vi "log analysis_gps.vi"() -> ()   [LabVIEW 2018] (continued)
0.0,0.000000000,0.000000000,\"631T\",11,3,3,3,04,00,20,00*7e5de74c\n\tsystem status\tnormal 2 27.700000 0 0\trobot status\t45.202909\t59.882712\t8.918700\t-0.461335\t0.674834\t-123.113809\t0.488000\t0.005000\n\t\n15:51:02.4\tlog_raw\tgps_raw\t#INSPVAXA,USB3,0,53.0,FINESTEERING,2107,283880.400,02000000,471d,15824;INS_ALIGNMENT_COMPLETE,INS_RTKFIXED,37.37066797060,126.72134375029,8.9215,22.3000,-0.3538,-0.2783,0.0388,-0.597615608,0.513014169,213.355161065,0.4357,0.3062,0.6023,0.1133,0.0940,0.0839,0.0973,0.1012,5.1494,0f000001,0*cddeff4e\n\tsystem status\tnormal 2 27.800000 0 0\trobot status\t45.054959\t59.684519\t8.921500\t-0.597616\t0.513014\t-123.355161\t0.488000\t-0.003000\n\t\n15:51:02.9\tlog_raw\tgps_raw\t#INSPVAXA,USB3,0,53.0,FINESTEERING,2107,283880.900,02000000,471d,15824;INS_ALIGNMENT_COMPLETE,INS_RTKFIXED,37.37066635165,126.72134221442,8.9278,22.3000,-0.3658,-0.2852,0.0396,-0.626245150,0.597396810,213.371902809,0.4357,0.3062,0.6023,0.1133,0.0940,0.0839,0.0973,0.1012,5.1494,0f000001,0*bdd5d949\n\tsystem status\tnormal 2 27.700000 0 0\trobot status\t44.918914\t59.504842\t8.927800\t-0.626245\t0.597397\t-123.371903\t0.492000\t0.000000\n\t\n15:51:03.4\tlog_raw\tgps_raw\t#DUALANTENNAHEADINGA,USB3,0,50.5,FINESTEERING,2107,283881.400,02000000,d426,15824;INSUFFICIENT_OBS,NONE,-1.000000000,0.000000000,0.000000000,0.0,0.000000000,0.000000000,\"631T\",11,3,3,3,04,00,20,00*4d958a84\n\tsystem status\tnormal 2 27.800000 0 0\trobot status\t44.773617\t59.313122\t8.931900\t-0.646552\t0.444640\t-123.445577\t0.501000\t0.006000\n\t\n15:51:03.9\tlog_raw\tgps_raw\t#INSPVAXA,USB3,0,50.5,FINESTEERING,2107,283881.900,02000000,471d,15824;INS_ALIGNMENT_COMPLETE,INS_RTKFIXED,37.37066299197,126.72133897955,8.9361,22.3000,-0.3474,-0.2868,0.0393,-0.593672744,0.610910921,213.511371032,0.4358,0.3048,0.6020,0.1139,0.0948,0.0841,0.0973,0.1012,5.1504,0f000001,0*060d8030\n\tsystem status\tnormal 2 27.700000 0 0\trobot status\t44.632374\t59.131970\t8.936100\t-0.593673\t0.610911\t-123.511371\t0.482000\t-0.001000\n\t\n15:51:04.4\tlog_raw\tgps_raw\t#DUALANTENNAHEADINGA,USB3,0,51.5,FINESTEERING,2107,283882.400,02000000,d426,15824;INSUFFICIENT_OBS,NONE,-1.000000000,0.000000000,0.000000000,0.0,0.000000000,0.000000000,\"631T\",12,3,3,3,04,00,20,00*3cefd7e2\n\tsystem status\tnormal 2 27.800000 0 0\trobot status\t44.487766\t58.944941\t8.939800\t-0.440117\t0.780812\t-123.484878\t0.511000\t0.000000\n\t\n15:51:04.9\tlog_raw\tgps_raw\t#INSPVAXA,USB3,0,51.5,FINESTEERING,2107,283882.900,02000000,471d,15824;INS_ALIGNMENT_COMPLETE,INS_RTKFIXED,37.37065963052,126.72133572900,8.9416,22.3000,-0.3499,-0.2875,0.0236,-0.546470396,0.861326947,213.517075808,0.4357,0.3040,0.6014,0.1142,0.0952,0.0840,0.0973,0.1012,5.1519,0f000001,0*24ce4552\n\tsystem status\tnormal 2 27.800000 0 0\trobot status\t44.344446\t58.758903\t8.941600\t-0.546470\t0.861327\t-123.517076\t0.491000\t-0.002000\n\t\n15:51:05.4\tlog_raw\tgps_raw\t#INSPVAXA,USB3,0,52.0,FINESTEERING,2107,283883.400,02000000,471d,15824;INS_ALIGNMENT_COMPLETE,INS_RTKFIXED,37.37065796164,126.72133411405,8.9451,22.3000,-0.3685,-0.2983,0.0398,-0.521036438,0.724479041,213.604247881,0.4353,0.3043,0.6007,0.1142,0.0953,0.0836,0.0972,0.1012,5.1533,0f000001,0*63d3ff51\n\tsystem status\tnormal 2 27.800000 0 0\trobot status\t44.201396\t58.573683\t8.945100\t-0.521036\t0.724479\t-123.604248\t0.493000\t-0.004000\n\t\n15:51:05.9\tlog_raw\tgps_raw\t#DUALANTENNAHEADINGA,USB3,0,52.0,FINESTEERING,2107,283883.900,02000000,d426,15824;INSUFFICIENT_OBS,NONE,-1.000000000,0.000000000,0.000000000,0.0,0.000000000,0.000000000,\"631T\",10,3,3,3,04,00,20,00*65cb768f\n\tsystem status\tnormal 2 27.800000 0 0\trobot status\t44.054708\t58.385576\t8.946000\t-0.360090\t0.706848\t-123.677696\t0.503000\t-0.011000\n\t\n15:51:06.4\tlog_raw\tgps_raw\t#DUALANTENNAHEADINGA,USB3,0,49.5,FINESTEERING,2107,283884.400,02000000,d426,15824;INSUFFICIENT_OBS,NONE,-1.000000000,0.000000000,0.000000000,0.0,0.000000000,0.000000000,\"631T\",9,3,3,3,04,00,20,00*1d3e0ccf\n\tsystem status\tnormal 2 27.800000 0 0\trobot status\t43.913169\t58.198898\t8.948900\t-0.506488\t0.685418\t-123.687701\t0.497000\t0.009000\n\t\n15:51:06.9\tlog_raw\tgps_raw\t#DUALANTENNAHEADINGA,USB3,0,49.5,FINESTEERING,2107,283884.900,02000000,d426,15824;INSUFFICIENT_OBS,NONE,-1.000000000,0.000000000,0.000000000,0.0,0.000000000,0.000000000,\"631T\",10,3,3,3,04,00,20,00*031e6964\n\tsystem status\tnormal 2 27.700000 0 0\trobot status\t43.771695\t58.014475\t8.953600\t-0.483140\t0.799105\t-123.568013\t0.566000\t-0.106000\n\t\n15:51:07.4\tlog_raw\tgps_raw\t#INSPVAXA,USB3,0,51.5,FINESTEERING,2107,283885.400,02000000,471d,15824;INS_ALIGNMENT_COMPLETE,INS_RTKFIXED,37.37065120654,126.72132762399,8.9567,22.3000,-0.3599,-0.3036,0.0416,-0.421250384,0.704031349,213.500996788,0.4347,0.3046,0.5988,0.1136,0.0944,0.0821,0.0969,0.1010,5.1559,0f000001,0*f6e8d8e3\n\tsystem status\tnormal 2 27.800000 0 0\trobot status\t43.626517\t57.823974\t8.956700\t-0.421250\t0.704031\t-123.500997\t0.476000\t0.038000\n\t\n15:51:07.9\tlog_raw\tgps_raw\t#DUALANTENNAHEADINGA,USB3,0,51.5,FINESTEERING,2107,283885.900,02000000,d426,15824;INSUFFICIENT_OBS,NONE,-1.000000000,0.000000000,0.000000000,0.0,0.000000000,0.000000000,\"631T\",9,3,3,3,04,00,20,00*45f2a281\n\tsystem status\tnormal 2 27.700000 0 0\trobot status\t43.483999\t57.637312\t8.961400\t-0.525632\t0.753190\t-123.406586\t0.428000\t0.092000\n\t\n15:51:08.4\tlog_raw\tgps_raw\t#DUALANTENNAHEADINGA,USB3,0,53.0,FINESTEERING,2107,283886.400,02000000,d426,15824;INSUFFICIENT_OBS,NONE,-1.000000000,0.000000000,0.000000000,0.0,0.000000000,0.000000000,\"631T\",9,3,3,3,04,00,20,00*f304b34d\n\tsystem status\tnormal 2 27.700000 0 0\trobot status\t43.341734\t57.449911\t8.964400\t-0.655210\t0.560645\t-123.324017\t0.473000\t0.021000\n\t\n15:51:08.9\tlog_raw\tgps_raw\t#DUALANTENNAHEADINGA,USB3,0,53.0,FINESTEERING,2107,283886.900,02000000,d426,15824;INSUFFICIENT_OBS,NONE,-1.000000000,0.000000000,0.000000000,0.0,0.000000000,0.000000000,\"631T\",9,3,3,3,04,00,20,00*6aeedf3b\n\tsystem status\tnormal 2 27.800000 0 0\trobot status\t43.199784\t57.262939\t8.968200\t-0.680653\t0.754053\t-123.210428\t0.466000\t0.053000\n\t\n15:51:09.4\tlog_raw\tgps_raw\t#DUALANTENNAHEADINGA,USB3,0,53.0,FINESTEERING,2107,283887.400,02000000,d426,15824;INSUFFICIENT_OBS,NONE,-1.000000000,0.000000000,0.000000000,0.0,0.000000000,0.000000000,\"631T\",9,3,3,3,04,00,20,00*f6e48158\n\tsystem status\tnormal 2 27.700000 0 0\trobot status\t43.057634\t57.072018\t8.971600\t-0.763083\t0.466087\t-123.102293\t0.415000\t0.111000\n\t\n15:51:09.9\tlog_raw\tgps_raw\t#DUALANTENNAHEADINGA,USB3,0,53.0,FINESTEERING,2107,283887.900,02000000,d426,15824;INSUFFICIENT_OBS,NONE,-1.000000000,0.000000000,0.000000000,0.0,0.000000000,0.000000000,\"631T\",9,3,3,3,04,00,20,00*6f0eed2e\n\tsystem status\tnormal 2 27.800000 0 0\trobot status\t42.915933\t56.883397\t8.974500\t-0.641098\t0.390257\t-123.007682\t0.428000\t0.084000\n\t\n15:51:10.4\tlog_raw\tgps_raw\t#DUALANTENNAHEADINGA,USB3,0,52.5,FINESTEERING,2107,283888.400,02000000,d426,15824;INSUFFICIENT_OBS,NONE,-1.000000000,0.000000000,0.000000000,0.0,0.000000000,0.000000000,\"631T\",10,3,3,3,04,00,20,00*e7048907\n\tsystem status\tnormal 2 27.700000 0 0\trobot status\t42.775640\t56.696889\t8.979100\t-0.681003\t0.747105\t-122.877604\t0.588000\t-0.127000\n\t\n15:51:10.9\tlog_raw\tgps_raw\t#DUALANTENNAHEADINGA,USB3,0,52.5,FINESTEERING,2107,283888.900,02000000,d426,15824;INSUFFICIENT_OBS,NONE,-1.000000000,0.000000000,0.000000000,0.0,0.000000000,0.000000000,\"631T\",10,3,3,3,04,00,20,00*5efbb762\n\tsystem status\tnormal 2 27.700000 0 0\trobot status\t42.634078\t56.507649\t8.981700\t-0.814755\t0.597074\t-122.710020\t0.592000\t-0.135000\n\t\n15:51:11.4\tlog_raw\tgps_raw\t#DUALANTENNAHEADINGA,USB3,0,46.0,FINESTEERING,2107,283889.400,02000000,d426,15824;INSUFFICIENT_OBS,NONE,-1.000000000,0.000000000,0.000000000,0.0,0.000000000,0.000000000,\"631T\",11,3,3,3,04,00,20,00*93f994bc\n\tsystem status\tnormal 2 27.700000 0 0\trobot status\t42.495049\t56.319089\t8.986300\t-0.601073\t0.725458\t-122.679569\t0.468000\t0.025000\n\t\n15:51:11.9\tlog_raw\tgps_raw\t#DUALANTENNAHEADINGA,USB3,0,46.0,FINESTEERING,2107,283889.900,02000000,d426,15824;INSUFFICIENT_OBS,NONE,-1.000000000,0.000000000,0.000000000,0.0,0.000000000,0.000000000,\"631T\",11,3,3,3,04,00,20,00*2a06aad9\n\tsystem status\tnormal 2 27.800000 0 0\trobot status\t42.353484\t56.121425\t8.991300\t-0.835162\t0.704682\t-122.703827\t0.503000\t-0.001000\n\t\n15:51:12.4\tlog_raw\tgps_raw\t#DUALANTENNAHEADINGA,USB3,0,49.5,FINESTEERING,2107,283890.400,02000000,d426,15824;INSUFFICIENT_OBS,NONE,-1.000000000,0.000000000,0.000000000,0.0,0.000000000,0.000000000,\"631T\",11,3,3,3,04,00,20,00*fe707008\n\tsystem status\tnormal 2 27.800000 0 0\trobot status\t42.214536\t55.932405\t8.994000\t-0.832597\t0.803383\t-122.691479\t0.495000\t-0.002000\n\t\n15:51:12.9\tlog_raw\tgps_raw\t#DUALANTENNAHEADINGA,USB3,0,49.5,FINESTEERING,2107,283890.900,02000000,d426,15824;INSUFFICIENT_OBS,NONE,-1.000000000,0.000000000,0.000000000,0.0,0.000000000,0.000000000,\"631T\",11,3,3,3,04,00,20,00*478f4e6d\n\tsystem status\tnormal 2 27.800000 0 0\trobot status\t42.072498\t55.741837\t8.997200\t-0.759363\t0.656487\t-122.762965\t0.579000\t-0.139000\n\t\n15:51:13.4\tlog_raw\tgps_raw\t#DUALANTENNAHEADINGA,USB3,0,50.5,FINESTEERING,2107,283891.400,02000000,d426,15824;INSUFFICIENT_OBS,NONE,-1.000000000,0.000000000,0.000000000,0.0,0.000000000,0.000000000,\"631T\",12,3,3,3,04,00,20,00*11a1be59\n\tsystem status\tnormal 2 27.700000 0 0\trobot status\t41.933995\t55.549806\t9.002300\t-0.915873\t0.288769\t-122.684066\t0.471000\t0.023000\n\t\n15:51:13.9\tlog_raw\tgps_raw\t#DUALANTENNAHEADINGA,USB3,0,50.5,FINESTEERING,2107,283891.900,02000000,d426,15824;INSUFFICIENT_OBS,NONE,-1.000000000,0.000000000,0.000000000,0.0,0.000000000,0.000000000,\"631T\",11,3,3,3,04,00,20,00*0b080695\n\tsystem status\tnormal 2 27.800000 0 0\trobot status\t41.790012\t55.354180\t9.005600\t-0.810761\t0.437065\t-122.626399\t0.585000\t-0.144000\n\t\n15:51:14.4\tlog_raw\tgps_raw\t#DUALANTENNAHEADINGA,USB3,0,51.0,FINESTEERING,2107,283892.400,02000000,d426,15824;INSUFFICIENT_OBS,NONE,-1.000000000,0.000000000,0.000000000,0.0,0.000000000,0.000000000,\"631T\",12,3,3,3,04,00,20,00*96f7835a\n\tsystem status\tnormal 2 27.800000 0 0\trobot status\t41.651158\t55.165638\t9.008000\t-0.628580\t0.466952\t-122.705405\t0.519000\t-0.026000\n\t\n15:51:14.9\tlog_raw\tgps_raw\t#DUALANTENNAHEADINGA,USB3,0,51.0,FINESTEERING,2107,283892.900,02000000,d426,15824;INSUFFICIENT_OBS,NONE,-1.000000000,0.000000000,0.000000000,0.0,0.000000000,0.000000000,\"631T\",11,3,3,3,04,00,20,00*8c5e3b96\n\tsystem status\tnormal 2 27.800000 0 0\trobot status\t41.510596\t54.974116\t9.012100\t-0.618825\t0.500579\t-122.716893\t0.486000\t0.000000\n\t\n15:51:15.4\tlog_raw\tgps_raw\t#DUALANTENNAHEADINGA,USB3,0,50.5,FINESTEERING,2107,283893.400,02000000,d426,15824;INSUFFICIENT_OBS,NONE,-1.000000000,0.000000000,0.000000000,0.0,0.000000000,0.000000000,\"631T\",12,3,3,3,04,00,20,00*ca11b7eb\n\tsystem status\tnormal 2 27.800000 0 0\trobot status\t41.369608\t54.781650\t9.014800\t-0.929782\t0.617797\t-122.679558\t0.590000\t-0.141000\n\t\n15:51:15.9\tlog_raw\tgps_raw\t#INSPVAXA,USB3,0,50.5,FINESTEERING,2107,283893.900,02000000,471d,15824;INS_ALIGNMENT_COMPLETE,INS_RTKFIXED,37.37062209490,126.72130052647,9.0192,22.3000,-0.3742,-0.3207,0.0346,-0.662095727,0.862366850,212.722532448,0.4356,0.3043,0.5955,0.1140,0.0944,0.0837,0.0963,0.1003,5.1649,0f000001,0*3a5d3b07\n\tsystem status\tnormal 2 27.800000 0 0\trobot status\t41.226263\t54.593043\t9.019200\t-0.662096\t0.862367\t-122.722532\t0.512000\t-0.016000\n\t\n15:51:16.4\tlog_raw\tgps_raw\t#DUALANTENNAHEADINGA,USB3,0,51.0,FINESTEERING,2107,283894.400,02008000,d426,15824;INSUFFICIENT_OBS,NONE,-1.000000000,0.000000000,0.000000000,0.0,0.000000000,0.000000000,\"631T\",13,3,3,3,04,00,20,00*e0279b34\n\tsystem status\tnormal 2 27.800000 0 0\trobot status\t41.087221\t54.406331\t9.023500\t-0.714306\t0.949922\t-122.700761\t0.488000\t0.028000\n\t\n15:51:16.9\tlog_raw\tgps_raw\t#DUALANTENNAHEADINGA,USB3,0,51.0,FINESTEERING,2107,283894.900,02008000,d426,15824;INSUFFICIENT_OBS,NONE,-1.000000000,0.000000000,0.000000000,0.0,0.000000000,0.000000000,\"631T\",14,3,3,3,04,00,20,00*13e62e1a\n\tsystem status\tnormal 2 27.800000 0 0\trobot status\t40.942985\t54.211235\t9.026200\t-0.826672\t0.663639\t-122.667749\t0.418000\t0.079000\n\t\n15:51:17.4\tlog_raw\tgps_raw\t#DUALANTENNAHEADINGA,USB3,0,51.0,FINESTEERING,2107,283895.400,02008000,d426,15824;INSUFFICIENT_OBS,NONE,-1.000000000,0.000000000,0.000000000,0.0,0.000000000,0.000000000,\"631T\",12,3,3,3,04,00,20,00*5a1d1fb5\n\tsystem status\tnormal 2 27.800000 0 0\trobot status\t40.798912\t54.016383\t9.030500\t-0.735055\t0.644417\t-122.767353\t0.515000\t-0.009000\n\t\n15:51:17.9\tlog_raw\tgps_raw\t#DUALANTENNAHEADINGA,USB3,0,51.0,FINESTEERING,2107,283895.900,02008000,d426,15824;INSUFFICIENT_OBS,NONE,-1.000000000,0.000000000,0.000000000,0.0,0.000000000,0.000000000,\"631T\",12,3,3,3,04,00,20,00*e3e221d0\n\tsystem status\tnormal 2 27.700000 0 0\trobot status\t40.659653\t53.826624\t9.034000\t-0.854452\t0.666010\t-122.702281\t0.516000\t0.013000\n\t\n15:51:18.4\tlog_raw\tgps_raw\t#DUALANTENNAHEADINGA,USB3,0,51.0,FINESTEERING,2107,283896.400,02008000,d426,15824;INSUFFICIENT_OBS,NONE,-1.000000000,0.000000000,0.000000000,0.0,0.000000000,0.000000000,\"631T\",10,3,3,3,04,00,20,00*98c1142f\n\tsystem status\tnormal 2 27.700000 0 0\trobot status\t40.518702\t53.636266\t9.036200\t-0.740829\t0.673835\t-122.581696\t0.455000\t0.058000\n\t\n15:51:18.9\tlog_raw\tgps_raw\t#DUALANTENNAHEADINGA,USB3,0,51.0,FINESTEERING,2107,283896.900,02008000,d426,15824;INSUFFICIENT_OBS,NONE,-1.000000000,0.000000000,0.000000000,0.0,0.000000000,0.000000000,\"631T\",10,3,3,3,04,00,20,00*213e2a4a\n\tsystem status\tnormal 2 27.800000 0 0\trobot status\t40.373143\t53.439598\t9.039600\t-0.643493\t0.780196\t-122.738509\t0.487000\t-0.009000\n\t\n15:51:19.4\tlog_raw\tgps_raw\t#DUALANTENNAHEADINGA,USB3,0,51.5,FINESTEERING,2107,283897.400,02008000,d426,15824;INSUFFICIENT_OBS,NONE,-1.000000000,0.000000000,0.000000000,0.0,0.000000000,0.000000000,\"631T\",10,3,3,3,04,00,20,00*a063f63a\n\tsystem status\tnormal 2 27.800000 0 0\trobot status\t40.234847\t53.245233\t9.043600\t-0.686027\t0.913912\t-122.740487\t0.438000\t0.106000\n\t\n15:51:19.9\tlog_raw\tgps_raw\t#DUALANTENNAHEADINGA,USB3,0,51.5,FINESTEERING,2107,283897.900,02008000,d426,15824;INSUFFICIENT_OBS,NONE,-1.000000000,0.000000000,0.000000000,0.0,0.000000000,0.000000000,\"631T\",10,3,3,3,04,00,20,00*199cc85f\n\tsystem status\tnormal 2 27.700000 0 0\trobot status\t40.098377\t53.053257\t9.046600\t-0.738622\t0.951323\t-122.581195\t0.499000\t-0.004000\n\t\n15:51:20.4\tlog_raw\tgps_raw\t#DUALANTENNAHEADINGA,USB3,0,52.5,FINESTEERING,2107,283898.400,02008000,d426,15824;INSUFFICIENT_OBS,NONE,-1.000000000,0.000000000,0.000000000,0.0,0.000000000,0.000000000,\"631T\",11,3,3,3,04,00,20,00*d9173f8a\n\tsystem status\tnormal 2 27.800000 0 0\trobot status\t39.959108\t52.857614\t9.048500\t-0.496098\t0.505815\t-122.625049\t0.536000\t-0.074000\n\t\n15:51:20.9\tlog_raw\tgps_raw\t#DUALANTENNAHEADINGA,USB3,0,52.5,FINESTEERING,2107,283898.900,02008000,d426,15824;INSUFFICIENT_OBS,NONE,-1.000000000,0.000000000,0.000000000,0.0,0.000000000,0.000000000,\"631T\",13,3,3,3,04,00,20,00*145c071e\n\tsystem status\tnormal 2 27.800000 0 0\trobot status\t39.819953\t52.658591\t9.052000\t-0.594721\t0.381164\t-122.648409\t0.487000\t-0.004000\n\t\n15:51:21.4\tlog_raw\tgps_raw\t#DUALANTENNAHEADINGA,USB3,0,50.5,FINESTEERING,2107,283899.400,02000000,d426,15824;INSUFFICIENT_OBS,NONE,-1.000000000,0.000000000,0.000000000,0.0,0.000000000,0.000000000,\"631T\",15,3,3,3,04,00,20,00*83bd1f58\n\tsystem status\tnormal 2 27.800000 0 0\trobot status\t39.682400\t52.462237\t9.055100\t-0.953666\t0.447596\t-122.714245\t0.499000\t-0.006000\n\t\n15:51:21.9\tlog_raw\tgps_raw\t#DUALANTENNAHEADINGA,USB3,0,50.5,FINESTEERING,2107,283899.900,02000000,d426,15824;INSUFFICIENT_OBS,NONE,-1.000000000,0.000000000,0.000000000,0.0,0.000000000,0.000000000,\"631T\",11,3,3,3,04,00,20,00*d32a2cdf\n\tsystem status\tnormal 2 27.800000 0 0\trobot status\t39.544744\t52.271556\t9.058700\t-0.891798\t0.472550\t-122.849537\t0.491000\t-0.012000\n\t\n15:51:22.4\tlog_raw\tgps_raw\t#DUALANTENNAHEADINGA,USB3,0,50.0,FINESTEERING,2107,283900.400,02000000,d426,15824;INSUFFICIENT_OBS,NONE,-1.000000000,0.000000000,0.000000000,0.0,0.000000000,0.000000000,\"631T\",9,3,3,3,04,00,20,00*b9862b26\n\tsystem status\tnormal 2 27.800000 0 0\trobot status\t39.405797\t52.077854\t9.062500\t-0.764089\t0.411472\t-122.863735\t0.496000\t-0.003000\n\t\n15:51:22.9\tlog_raw\tgps_raw\t#DUALANTENNAHEADINGA,USB3,0,50.0,FINESTEERING,2107,283900.900,02000000,d426,15824;INSUFFICIENT_OBS,NONE,-1.000000000,0.000000000,0.000000000,0.0,0.000000000,0.000000000,\"631T\",9,3,3,3,04,00,20,00*206c4750\n\tsystem status\tnormal 2 27.800000 0 0\trobot status\t39.267771\t51.887049\t9.063700\t-0.797925\t0.282796\t-122.902803\t0.497000\t-0.007000\n\t\n15:51:23.4\tlog_raw\tgps_raw\t#DUALANTENNAHEADINGA,USB3,0,50.0,FINESTEERING,2107,283901.400,02008000,d426,15824;INSUFFICIENT_OBS,NONE,-1.000000000,0.000000000,0.000000000,0.0,0.000000000,0.000000000,\"631T\",9,3,3,3,04,00,20,00*432dfdec\n\tsystem status\tnormal 2 27.800000 0 0\trobot status\t39.128381\t51.693559\t9.066000\t-0.719639\t0.206522\t-123.010548\t0.486000\t-0.005000\n\t\n15:51:23.9\tlog_raw\tgps_raw\t\tsystem status\tnormal 2 27.800000 0 0\trobot status\t38.989994\t51.499767\t9.067300\t-0.777600\t0.277803\t-123.030098\t0.499000\t-0.005000\n\t\n15:51:24.4\tlog_raw\tgps_raw\t#DUALANTENNAHEADINGA,USB3,0,50.0,FINESTEERING,2107,283902.400,02008000,d426,15824;INSUFFICIENT_OBS,NONE,-1.000000000,0.000000000,0.000000000,0.0,0.000000000,0.000000000,\"631T\",11,3,3,3,04,00,20,00*7952b8b1\n\tsystem status\tnormal 2 27.800000 0 0\trobot status\t38.850935\t51.307304\t9.068500\t-0.688010\t0.215505\t-123.058132\t0.490000\t-0.004000\n\t\n15:51:24.9\tlog_raw\tgps_raw\t#DUALANTENNAHEADINGA,USB3,0,50.0,FINESTEERING,2107,283902.900,02008000,d426,15824;INSUFFICIENT_OBS,NONE,-1.000000000,0.000000000,0.000000000,0.0,0.000000000,0.000000000,\"631T\",10,3,3,3,04,00,20,00*174f068c\n\tsystem status\tnormal 2 27.800000 0 0\trobot status\t38.711980\t51.114729\t9.069000\t-0.641697\t0.148527\t-123.181965\t0.483000\t-0.006000\n\t\n15:51:25.4\tlog_raw\tgps_raw\t#INSPVAXA,USB3,0,49.0,FINESTEERING,2107,283903.450,02008000,471d,15824;INS_ALIGNMENT_COMPLETE,INS_RTKFIXED,37.37058884071,126.72127040415,9.0705,22.3000,-0.3807,-0.3020,0.0207,-0.679787264,0.064920800,213.254026909,0.4334,0.3029,0.5969,0.1133,0.0944,0.0822,0.0966,0.1006,5.1769,0f000001,0*71c893b5\n\tsystem status\tnormal 2 27.800000 0 0\trobot status\t38.558078\t50.902353\t9.070500\t-0.679787\t0.064921\t-123.254027\t0.491000\t0.000000\n\t\n15:51:25.9\tlog_raw\tgps_raw\t\tsystem status\tnormal 2 27.800000 0 0\trobot status\t38.430780\t50.728191\t9.070500\t-0.714844\t0.073949\t-123.369053\t0.507000\t-0.006000\n\t\n15:51:26.4\tlog_raw\tgps_raw\t#DUALANTENNAHEADINGA,USB3,0,48.5,FINESTEERING,2107,283904.400,02008000,d426,15824;INSUFFICIENT_OBS,NONE,-1.000000000,0.000000000,0.000000000,0.0,0.000000000,0.000000000,\"631T\",11,3,3,3,04,00,20,00*de92d86f\n\tsystem status\tnormal 2 27.800000 0 0\trobot status\t38.290244\t50.540108\t9.070000\t-0.537424\t0.083817\t-123.460218\t0.505000\t-0.001000\n\t\n15:51:26.9\tlog_raw\tgps_raw\t#INSPVAXA,USB3,0,48.5,FINESTEERING,2107,283904.950,02008000,471d,15824;INS_ALIGNMENT_COMPLETE,INS_RTKFIXED,37.37058369457,126.72126562815,9.0689,22.3000,-0.3526,-0.2989,0.0165,-0.611939006,0.199763029,213.494948606,0.4333,0.3029,0.5964,0.1131,0.0941,0.0816,0.0965,0.1006,5.1782,0f000001,0*4f2b9d43\n\tsystem status\tnormal 2 27.800000 0 0\trobot status\t38.135027\t50.331212\t9.068900\t-0.611939\t0.199763\t-123.494949\t0.488000\t0.002000\n\t\n15:51:27.4\tlog_raw\tgps_raw\t#DUALANTENNAHEADINGA,USB3,0,51.0,FINESTEERING,2107,283905.400,02000000,d426,15824;INSUFFICIENT_OBS,NONE,-1.000000000,0.000000000,0.000000000,0.0,0.000000000,0.000000000,\"631T\",11,3,3,3,04,00,20,00*d1fcf2fa\n\tsystem status\tnormal 2 27.800000 0 0\trobot status\t38.008015\t50.160168\t9.069500\t-0.542039\t0.521340\t-123.552730\t0.510000\t-0.008000\n\t\n15:51:27.9\tlog_raw\tgps_raw\t#INSPVAXA,USB3,0,51.0,FINESTEERING,2107,283905.950,02000000,471d,15824;INS_ALIGNMENT_COMPLETE,INS_RTKFIXED,37.37058025923,126.72126241939,9.0707,22.3000,-0.3812,-0.3080,0.0278,-0.525044361,0.591334106,213.674985050,0.4335,0.3031,0.5959,0.1142,0.0952,0.0829,0.0965,0.1005,5.1795,0f000001,0*069603aa\n\tsystem status\tnormal 2 27.800000 0 0\trobot status\t37.850801\t49.949944\t9.070700\t-0.525044\t0.591334\t-123.674985\t0.490000\t-0.010000\n\t\n15:51:28.4\tlog_raw\tgps_raw\t#DUALANTENNAHEADINGA,USB3,0,50.0,FINESTEERING,2107,283906.400,02000000,d426,15824;INSUFFICIENT_OBS,NONE,-1.000000000,0.000000000,0.000000000,0.0,0.000000000,0.000000000,\"631T\",11,3,3,3,04,00,20,00*03d02935\n\tsystem status\tnormal 2 27.800000 0 0\trobot status\t37.721666\t49.778721\t9.072000\t-0.766758\t0.222071\t-123.821998\t0.498000\t0.002000\n\t\n15:51:28.9\tlog_raw\tgps_raw\t#INSPVAXA,USB3,0,50.0,FINESTEERING,2107,283906.950,02000000,471d,15824;INS_ALIGNMENT_COMPLETE,INS_RTKFIXED,37.37057686520,126.72125915274,9.0748,22.3000,-0.3835,-0.3158,0.0154,-0.714794692,0.316524554,214.061130278,0.4338,0.3036,0.5955,0.1138,0.0946,0.0824,0.0964,0.1005,5.1810,0f000001,0*ecb7aa1d\n\tsystem status\tnormal 2 27.800000 0 0\trobot status\t37.561446\t49.573260\t9.074800\t-0.714795\t0.316525\t-124.061130\t0.487000\t-0.014000\n\t\n15:51:29.4\tlog_raw\tgps_raw\t#DUALANTENNAHEADINGA,USB3,0,51.0,FINESTEERING,2107,283907.400,02000000,d426,15824;INSUFFICIENT_OBS,NONE,-1.000000000,0.000000000,0.000000000,0.0,0.000000000,0.000000000,\"631T\",12,3,3,3,04,00,20,00*a91a7de1\n\tsystem status\tnormal 2 27.800000 0 0\trobot status\t37.431645\t49.403463\t9.075400\t-0.727763\t0.386272\t-124.115963\t0.497000\t-0.002000\n\t\n15:51:29.9\tlog_raw\tgps_raw\t#DUALANTENNAHEADINGA,USB3,0,51.0,FINESTEERING,2107,283907.900,02000000,d426,15824;INSUFFICIENT_OBS,NONE,-1.000000000,0.000000000,0.000000000,0.0,0.000000000,0.000000000,\"631T\",11,3,3,3,04,00,20,00*b3b3c52d\n\tsystem status\tnormal 2 27.800000 0 0\trobot status\t37.285960\t49.213886\t9.077100\t-0.681823\t0.666598\t-124.183643\t0.489000\t0.000000\n\t\n15:51:30.4\tlog_raw\tgps_raw\t\tsystem status\tnormal 2 27.800000 0 0\trobot status\t37.139701\t49.021968\t9.079900\t-0.693107\t0.423783\t-124.359573\t0.494000\t-0.014000\n\t\n15:51:30.9\tlog_raw\tgps_raw\t#DUALANTENNAHEADINGA,USB3,0,52.5,FINESTEERING,2107,283908.900,02000000,d426,15824;INSUFFICIENT_OBS,NONE,-1.000000000,0.000000000,0.000000000,0.0,0.000000000,0.000000000,\"631T\",11,3,3,3,04,00,20,00*485f6a09\n\tsystem status\tnormal 2 27.800000 0 0\trobot status\t36.994621\t48.833861\t9.081200\t-0.669847\t0.417927\t-124.429930\t0.505000\t-0.003000\n\t\n15:51:31.4\tlog_raw\tgps_raw\t#DUALANTENNAHEADINGA,USB3,0,50.5,FINESTEERING,2107,283909.400,02000000,d426,15824;INSUFFICIENT_OBS,NONE,-1.000000000,0.000000000,0.000000000,0.0,0.000000000,0.000000000,\"631T\",12,3,3,3,04,00,20,00*f7a77b54\n\tsystem status\tnormal 2 27.700000 0 0\trobot status\t36.850603\t48.648977\t9.083400\t-0.538230\t0.514884\t-124.422751\t0.508000\t0.003000\n\t\n15:51:31.9\tlog_raw\tgps_raw\t#DUALANTENNAHEADINGA,USB3,0,50.5,FINESTEERING,2107,283909.900,02000000,d426,15824;INSUFFICIENT_OBS,NONE,-1.000000000,0.000000000,0.000000000,0.0,0.000000000,0.000000000,\"631T\",13,3,3,3,04,00,20,00*99bac569\n\tsystem status\tnormal 2 27.800000 0 0\trobot status\t36.703464\t48.458985\t9.085500\t-0.467392\t0.376100\t-124.487346\t0.505000\t-0.002000\n\t\n15:51:32.4\tlog_raw\tgps_raw\t#INSPVAXA,USB3,0,48.0,FINESTEERING,2107,283910.450,02000000,471d,15824;INS_ALIGNMENT_COMPLETE,INS_RTKFIXED,37.37056496909,126.72124764665,9.0863,22.3000,-0.3554,-0.3247,0.0202,-0.305074143,0.317241831,214.523867584,0.4346,0.3048,0.5954,0.1134,0.0941,0.0823,0.0963,0.1003,5.1868,0f000001,0*02f445bc\n\tsystem status\tnormal 2 27.800000 0 0\trobot status\t36.542256\t48.252979\t9.086300\t-0.305074\t0.317242\t-124.523868\t0.490000\t0.003000\n\t\n15:51:32.9\tlog_raw\tgps_raw\t#DUALANTENNAHEADINGA,USB3,0,48.0,FINESTEERING,2107,283910.900,02000000,d426,15824;INSUFFICIENT_OBS,NONE,-1.000000000,0.000000000,0.000000000,0.0,0.000000000,0.000000000,\"631T\",12,3,3,3,04,00,20,00*14a1a59f\n\tsystem status\tnormal 2 27.700000 0 0\trobot status\t36.411411\t48.084639\t9.088200\t-0.392519\t0.181008\t-124.498540\t0.481000\t0.036000\n\t\n15:51:33.4\tlog_raw\tgps_raw\t#INSPVAXA,USB3,0,49.5,FINESTEERING,2107,283911.450,02000000,471d,15824;INS_ALIGNMENT_COMPLETE,INS_RTKFIXED,37.37056161289,126.72124438523,9.0878,22.3000,-0.3391,-0.2889,0.0305,-0.373763892,0.193972280,214.477350215,0.4341,0.3042,0.5952,0.1138,0.0946,0.0829,0.0963,0.1003,5.1884,0f000001,0*19e64a77\n\tsystem status\tnormal 2 27.800000 0 0\trobot status\t36.253364\t47.880494\t9.087800\t-0.373764\t0.193972\t-124.477350\t0.404000\t0.102000\n\t\n15:51:33.9\tlog_raw\tgps_raw\t\tsystem status\tnormal 2 27.700000 0 0\trobot status\t36.123317\t47.713233\t9.089300\t-0.360632\t0.314801\t-124.348326\t0.459000\t0.057000\n\t\n15:51:34.4\tlog_raw\tgps_raw\t#DUALANTENNAHEADINGA,USB3,0,51.0,FINESTEERING,2107,283912.400,02000000,d426,15824;INSUFFICIENT_OBS,NONE,-1.000000000,0.000000000,0.000000000,0.0,0.000000000,0.000000000,\"631T\",10,3,3,3,04,00,20,00*2305d898\n\tsystem status\tnormal 2 27.700000 0 0\trobot status\t35.979477\t47.532926\t9.091500\t-0.119003\t0.863195\t-124.217605\t0.439000\t0.098000\n\t\n15:51:34.9\tlog_raw\tgps_raw\t#INSPVAXA,USB3,0,51.0,FINESTEERING,2107,283912.950,02000000,471d,15824;INS_ALIGNMENT_COMPLETE,INS_RTKFIXED,37.37055667019,126.72123951954,9.0936,22.3000,-0.3847,-0.3125,0.0281,-0.432078717,0.899277400,214.193265396,0.4336,0.3036,0.5951,0.1137,0.0947,0.0831,0.0963,0.1003,5.1898,0f000001,0*1102a532\n\tsystem status\tnormal 2 27.700000 0 0\trobot status\t35.822370\t47.331932\t9.093600\t-0.432079\t0.899277\t-124.193265\t0.468000\t0.059000\n\t\n15:51:35.4\tlog_raw\tgps_raw\t#DUALANTENNAHEADINGA,USB3,0,52.5,FINESTEERING,2107,283913.400,02000000,d426,15824;INSUFFICIENT_OBS,NONE,-1.000000000,0.000000000,0.000000000,0.0,0.000000000,0.000000000,\"631T\",11,3,3,3,04,00,20,00*6088c139\n\tsystem status\tnormal 2 27.700000 0 0\trobot status\t35.693456\t47.170033\t9.096300\t-0.270486\t0.808496\t-124.053273\t0.471000\t0.026000\n\t\n15:51:35.9\tlog_raw\tgps_raw\t#DUALANTENNAHEADINGA,USB3,0,52.5,FINESTEERING,2107,283913.900,02000000,d426,15824;INSUFFICIENT_OBS,NONE,-1.000000000,0.000000000,0.000000000,0.0,0.000000000,0.000000000,\"631T\",13,3,3,3,04,00,20,00*adc3f9ad\n\tsystem status\tnormal 2 27.700000 0 0\trobot status\t35.548769\t46.987396\t9.101900\t-0.258178\t0.897481\t-123.945231\t0.418000\t0.087000\n\t\n15:51:36.4\tlog_raw\tgps_raw\t#INSPVAXA,USB3,0,48.0,FINESTEERING,2107,283914.450,02000000,471d,15824;INS_ALIGNMENT_COMPLETE,INS_RTKFIXED,37.37055172372,126.72123465908,9.1045,22.3000,-0.3321,-0.3029,0.0193,-0.498508011,0.792000262,213.719525231,0.4335,0.3037,0.5952,0.1132,0.0940,0.0823,0.0963,0.1003,5.1929,0f000001,0*c17a4193\n\tsystem status\tnormal 2 27.700000 0 0\trobot status\t35.391838\t46.782952\t9.104500\t-0.498508\t0.792000\t-123.719525\t0.476000\t0.038000\n\t\n15:51:36.9\tlog_raw\tgps_raw\t#INSPVAXA,USB3,0,48.0,FINESTEERING,2107,283914.950,02000000,471d,15824;INS_ALIGNMENT_COMPLETE,INS_RTKFIXED,37.37055006660,126.72123300626,9.1068,22.3000,-0.3507,-0.2983,0.0012,-0.233266820,0.708375211,213.616604793,0.4335,0.3037,0.5952,0.1132,0.0940,0.0823,0.0963,0.1003,5.1929,0f000001,0*8c718c31\n\tsystem status\tnormal 2 27.700000 0 0\trobot status\t35.245434\t46.599038\t9.106800\t-0.233267\t0.708375\t-123.616605\t0.594000\t-0.145000\n\t\n15:51:37.4\tlog_raw\tgps_raw\t#DUALANTENNAHEADINGA,USB3,0,47.0,FINESTEERING,2107,283915.400,02000000,d426,15824;INSUFFICIENT_OBS,NONE,-1.000000000,0.000000000,0.000000000,0.0,0.000000000,0.000000000,\"631T\",11,3,3,3,04,00,20,00*7daa9230\n\tsystem status\tnormal 2 27.700000 0 0\trobot status\t35.118694\t46.432744\t9.110300\t-0.354394\t0.687175\t-123.470230\t0.444000\t0.087000\n\t\n15:51:37.9\tlog_raw\tgps_raw\t#INSPVAXA,USB3,0,47.0,FINESTEERING,2107,283915.950,02000000,471d,15824;INS_ALIGNMENT_COMPLETE,INS_RTKFIXED,37.37054673087,126.72122978879,9.1114,22.3000,-0.3591,-0.2902,0.0351,-0.280063258,0.768282729,213.379617811,0.4334,0.3035,0.5951,0.1128,0.0937,0.0818,0.0963,0.1003,5.1943,0f000001,0*df737fc9\n\tsystem status\tnormal 2 27.700000 0 0\trobot status\t34.960436\t46.228825\t9.111400\t-0.280063\t0.768283\t-123.379618\t0.408000\t0.106000\n\t\n15:51:38.4\tlog_raw\tgps_raw\t#INSPVAXA,USB3,0,49.0,FINESTEERING,2107,283916.450,02000000,471d,15824;INS_ALIGNMENT_COMPLETE,INS_RTKFIXED,37.37054503635,126.72122820634,9.1136,22.3000,-0.3595,-0.2800,0.0167,-0.568627617,0.574232692,213.297475739,0.4336,0.3033,0.5948,0.1126,0.0935,0.0813,0.0963,0.1003,5.1956,0f000001,0*cacfced8\n\tsystem status\tnormal 2 27.700000 0 0\trobot status\t34.820265\t46.040760\t9.113600\t-0.568628\t0.574233\t-123.297476\t0.435000\t0.085000\n\t\n15:51:38.9\tlog_raw\tgps_raw\t#INSPVAXA,USB3,0,49.0,FINESTEERING,2107,283916.950,02000000,471d,15824;INS_ALIGNMENT_COMPLETE,INS_RTKFIXED,37.37054332182,126.72122657762,9.1146,22.3000,-0.3450,-0.3025,0.0148,-0.530748763,0.232275373,213.084868526,0.4336,0.3033,0.5948,0.1126,0.0935,0.0813,0.0963,0.1003,5.1956,0f000001,0*d44f9e4e\n\tsystem status\tnormal 2 27.800000 0 0\trobot status\t34.675995\t45.850474\t9.114600\t-0.530749\t0.232275\t-123.084869\t0.426000\t0.090000\n\t\n15:51:39.4\tlog_raw\tgps_raw\t#INSPVAXA,USB3,0,49.0,FINESTEERING,2107,283917.450,02000000,471d,15824;INS_ALIGNMENT_COMPLETE,INS_RTKFIXED,37.37054163352,126.72122501811,9.1165,22.3000,-0.3554,-0.2975,0.0340,-0.824959720,0.443504930,213.062065508,0.4333,0.3029,0.5945,0.1125,0.0935,0.0809,0.0963,0.1003,5.1969,0f000001,0*c7e22c84\n\tsystem status\tnormal 2 27.700000 0 0\trobot status\t34.537857\t45.663099\t9.116500\t-0.824960\t0.443505\t-123.062066\t0.432000\t0.112000\n\t\n15:51:39.9\tlog_raw\tgps_raw\t\tsystem status\tnormal 2 27.700000 0 0\trobot status\t34.412531\t45.498188\t9.117800\t-0.605490\t0.332232\t-122.930171\t0.590000\t-0.128000\n\t\n15:51:40.4\tlog_raw\tgps_raw\t#DUALANTENNAHEADINGA,USB3,0,50.5,FINESTEERING,2107,283918.400,02000000,d426,15824;INSUFFICIENT_OBS,NONE,-1.000000000,0.000000000,0.000000000,0.0,0.000000000,0.000000000,\"631T\",9,3,3,3,04,00,20,00*849f5ce0\n\tsystem status\tnormal 2 27.700000 0 0\trobot status\t34.271777\t45.309013\t9.120100\t-0.535046\t0.464441\t-122.778871\t0.425000\t0.084000\n\t\n15:51:40.9\tlog_raw\tgps_raw\t#INSPVAXA,USB3,0,50.5,FINESTEERING,2107,283918.950,02000000,471d,15824;INS_ALIGNMENT_COMPLETE,INS_RTKFIXED,37.37053657031,126.72122025773,9.1231,22.3000,-0.3626,-0.3082,0.0292,-0.664128587,0.419081296,212.844872537,0.4329,0.3028,0.5939,0.1124,0.0937,0.0805,0.0963,0.1003,5.1982,0f000001,0*4b642c0a\n\tsystem status\tnormal 2 27.700000 0 0\trobot status\t34.116190\t45.101162\t9.123100\t-0.664129\t0.419081\t-122.844873\t0.590000\t-0.139000\n\t\n15:51:41.4\tlog_raw\tgps_raw\t#INSPVAXA,USB3,0,47.0,FINESTEERING,2107,283919.450,02000000,471d,15824;INS_ALIGNMENT_COMPLETE,INS_RTKFIXED,37.37053487627,126.72121868660,9.1237,22.3000,-0.3564,-0.3030,0.0002,-0.479328708,0.369667523,212.741899400,0.4326,0.3022,0.5934,0.1124,0.0936,0.0802,0.0962,0.1003,5.1992,0f000001,0*77fc8fa5\n\tsystem status\tnormal 2 27.800000 0 0\trobot status\t33.977022\t44.913151\t9.123700\t-0.479329\t0.369668\t-122.741899\t0.563000\t-0.095000\n\t\n15:51:41.9\tlog_raw\tgps_raw\t#INSPVAXA,USB3,0,47.0,FINESTEERING,2107,283919.950,02000000,471d,15824;INS_ALIGNMENT_COMPLETE,INS_RTKFIXED,37.37053314698,126.72121706257,9.1241,22.3000,-0.3522,-0.3058,0.0197,-0.363383073,0.096459549,212.853457646,0.4326,0.3022,0.5934,0.1124,0.0936,0.0802,0.0962,0.1003,5.1992,0f000001,0*a718023e\n\tsystem status\tnormal 2 27.800000 0 0\trobot status\t33.833168\t44.721227\t9.124100\t-0.363383\t0.096460\t-122.853458\t0.509000\t-0.006000\n\t\n15:51:42.4\tlog_raw\tgps_raw\t#INSPVAXA,USB3,0,52.0,FINESTEERING,2107,283920.450,02000000,471d,15824;INS_ALIGNMENT_COMPLETE,INS_RTKFIXED,37.37053146524,126.72121553588,9.1258,22.3000,-0.3500,-0.2976,0.0272,-0.521767170,0.221904426,212.799458593,0.4324,0.3020,0.5928,0.1125,0.0936,0.0799,0.0961,0.1002,5.2000,0f000001,0*115d72dc\n\tsystem status\tnormal 2 27.700000 0 0\trobot status\t33.697936\t44.534580\t9.125800\t-0.521767\t0.221904\t-122.799459\t0.467000\t0.019000\n\t\n15:51:42.9\tlog_raw\tgps_raw\t\tsystem status\tnormal 2 27.800000 0 0\trobot status\t33.570790\t44.360046\t9.127600\t-0.416671\t0.264015\t-122.836790\t0.496000\t0.000000\n\t\n15:51:43.4\tlog_raw\tgps_raw\t#INSPVAXA,USB3,0,48.0,FINESTEERING,2107,283921.450,02000000,471d,15824;INS_ALIGNMENT_COMPLETE,INS_RTKFIXED,37.37052802282,126.72121240001,9.1291,22.3000,-0.3507,-0.3057,0.0251,-0.215783432,0.396063272,212.883809512,0.4322,0.3017,0.5920,0.1125,0.0935,0.0797,0.0960,0.1002,5.2006,0f000001,0*28d97cd1\n\tsystem status\tnormal 2 27.800000 0 0\trobot status\t33.420166\t44.152525\t9.129100\t-0.215783\t0.396063\t-122.883810\t0.498000\t-0.006000\n\t\n15:51:43.9\tlog_raw\tgps_raw\t#INSPVAXA,USB3,0,48.0,FINESTEERING,2107,283921.950,02000000,471d,15824;INS_ALIGNMENT_COMPLETE,INS_RTKFIXED,37.37052634631,126.72121089774,9.1341,22.3000,-0.3596,-0.2838,0.0323,-0.415372337,0.706980969,212.926580959,0.4322,0.3017,0.5920,0.1125,0.0935,0.0797,0.0960,0.1002,5.2006,0f000001,0*148fe8d6\n\tsystem status\tnormal 2 27.800000 0 0\trobot status\t33.287097\t43.966459\t9.134100\t-0.415372\t0.706981\t-122.926581\t0.502000\t-0.004000\n\t\n15:51:44.4\tlog_raw\tgps_raw\t#INSPVAXA,USB3,0,43.0,FINESTEERING,2107,283922.450,02000000,471d,15824;INS_ALIGNMENT_COMPLETE,INS_RTKFIXED,37.37052460357,126.72120933072,9.1390,22.3000,-0.3446,-0.3015,0.0137,-0.382873007,0.563010953,212.928415689,0.4322,0.3018,0.5913,0.1124,0.0934,0.0795,0.0959,0.1001,5.2012,0f000001,0*06ecfb60\n\tsystem status\tnormal 2 27.800000 0 0\trobot status\t33.148293\t43.773042\t9.139000\t-0.382873\t0.563011\t-122.928416\t0.500000\t0.004000\n\t\n15:51:44.9\tlog_raw\tgps_raw\t#INSPVAXA,USB3,0,43.0,FINESTEERING,2107,283922.950,02000000,471d,15824;INS_ALIGNMENT_COMPLETE,INS_RTKFIXED,37.37052292197,126.72120779195,9.1447,22.3000,-0.3494,-0.2921,0.0334,-0.254339897,0.526441587,212.988420393,0.4322,0.3018,0.5913,0.1124,0.0934,0.0795,0.0959,0.1001,5.2012,0f000001,0*74466e11\n\tsystem status\tnormal 2 27.800000 0 0\trobot status\t33.011992\t43.586411\t9.144700\t-0.254340\t0.526442\t-122.988420\t0.484000\t-0.010000\n\t\n15:51:45.4\tlog_raw\tgps_raw\t#INSPVAXA,USB3,0,45.5,FINESTEERING,2107,283923.450,02000000,471d,15824;INS_ALIGNMENT_COMPLETE,INS_RTKFIXED,37.37052118554,126.72120621046,9.1491,22.3000,-0.3583,-0.2946,0.0183,-0.080875673,0.518402555,213.021069152,0.4321,0.3020,0.5906,0.1124,0.0934,0.0794,0.0958,0.1001,5.2021,0f000001,0*09f1c4be\n\tsystem status\tnormal 2 27.800000 0 0\trobot status\t32.871906\t43.393695\t9.149100\t-0.080876\t0.518403\t-123.021069\t0.504000\t-0.001000\n\t\n15:51:45.9\tlog_raw\tgps_raw\t#INSPVAXA,USB3,0,45.5,FINESTEERING,2107,283923.950,02000000,471d,15824;INS_ALIGNMENT_COMPLETE,INS_RTKFIXED,37.37051949937,126.72120468984,9.1523,22.3000,-0.3577,-0.2933,0.0036,-0.207836211,0.548820152,213.042486887,0.4321,0.3020,0.5906,0.1124,0.0934,0.0794,0.0958,0.1001,5.2021,0f000001,0*e62c9616\n\tsystem status\tnormal 2 27.700000 0 0\trobot status\t32.737212\t43.206556\t9.152300\t-0.207836\t0.548820\t-123.042487\t0.497000\t0.001000\n\t\n15:51:46.4\tlog_raw\tgps_raw\t#INSPVAXA,USB3,0,50.0,FINESTEERING,2107,283924.450,02000000,471d,15824;INS_ALIGNMENT_COMPLETE,INS_RTKFIXED,37.37051776431,126.72120311911,9.1553,22.3000,-0.3480,-0.2880,0.0361,-0.209670609,0.595606109,213.112162287,0.4321,0.3024,0.5900,0.1124,0.0933,0.0793,0.0957,0.1000,5.2033,0f000001,0*9cc91f60\n\tsystem status\tnormal 2 27.800000 0 0\trobot status\t32.598079\t43.013992\t9.155300\t-0.209671\t0.595606\t-123.112162\t0.483000\t-0.003000\n\t\n15:51:46.9\tlog_raw\tgps_raw\t#INSPVAXA,USB3,0,50.0,FINESTEERING,2107,283924.950,02000000,471d,15824;INS_ALIGNMENT_COMPLETE,INS_RTKFIXED,37.37051602540,126.72120154897,9.1565,22.3000,-0.3460,-0.2879,0.0300,-0.302016421,0.742841362,213.157571504,0.4321,0.3024,0.5900,0.1124,0.0933,0.0793,0.0957,0.1000,5.2033,0f000001,0*c2c8a9b5\n\tsystem status\tnormal 2 27.800000 0 0\trobot status\t32.458999\t42.821000\t9.156500\t-0.302016\t0.742841\t-123.157572\t0.483000\t0.004000\n\t\n15:51:47.4\tlog_raw\tgps_raw\t#INSPVAXA,USB3,0,50.5,FINESTEERING,2107,283925.450,02000000,471d,15824;INS_ALIGNMENT_COMPLETE,INS_RTKFIXED,37.37051431661,126.72119998698,9.1612,22.3000,-0.3602,-0.3017,0.0078,-0.150276510,0.673330770,213.275693569,0.4320,0.3027,0.5895,0.1123,0.0933,0.0792,0.0956,0.1000,5.2048,0f000001,0*406b8736\n\tsystem status\tnormal 2 27.700000 0 0\trobot status\t32.320640\t42.631352\t9.161200\t-0.150277\t0.673331\t-123.275694\t0.499000\t-0.003000\n\t\n15:51:47.9\tlog_raw\tgps_raw\t#INSPVAXA,USB3,0,50.5,FINESTEERING,2107,283925.950,02000000,471d,15824;INS_ALIGNMENT_COMPLETE,INS_RTKFIXED,37.37051260472,126.72119841122,9.1660,22.3000,-0.3548,-0.3097,0.0154,-0.098276795,0.507978734,213.441186851,0.4320,0.3027,0.5895,0.1123,0.0933,0.0792,0.0956,0.1000,5.2048,0f000001,0*9b14382d\n\tsystem status\tnormal 2 27.800000 0 0\trobot status\t32.181062\t42.441359\t9.166000\t-0.098277\t0.507979\t-123.441187\t0.492000\t-0.014000\n\t\n15:51:48.4\tlog_raw\tgps_raw\t#DUALANTENNAHEADINGA,USB3,0,48.5,FINESTEERING,2107,283926.400,02000000,d426,15824;INSUFFICIENT_OBS,NONE,-1.000000000,0.000000000,0.000000000,0.0,0.000000000,0.000000000,\"631T\",10,3,3,3,04,00,20,00*e1e7b78d\n\tsystem status\tnormal 2 27.800000 0 0\trobot status\t32.053906\t42.269246\t9.169900\t-0.190863\t0.556821\t-123.603158\t0.484000\t-0.014000\n\t\n15:51:48.9\tlog_raw\tgps_raw\t#INSPVAXA,USB3,0,48.5,FINESTEERING,2107,283926.950,02000000,471d,15824;INS_ALIGNMENT_COMPLETE,INS_RTKFIXED,37.37050917237,126.72119519528,9.1767,22.3000,-0.3519,-0.3025,0.0208,-0.173094935,0.655730796,213.776498687,0.4320,0.3032,0.5892,0.1131,0.0942,0.0804,0.0956,0.0999,5.2064,0f000001,0*f79ccc8c\n\tsystem status\tnormal 2 27.700000 0 0\trobot status\t31.896199\t42.060422\t9.176700\t-0.173095\t0.655731\t-123.776499\t0.497000\t0.000000\n\t\n15:51:49.4\tlog_raw\tgps_raw\t#INSPVAXA,USB3,0,45.5,FINESTEERING,2107,283927.450,02000000,471d,15824;INS_ALIGNMENT_COMPLETE,INS_RTKFIXED,37.37050743516,126.72119359440,9.1795,22.3000,-0.3580,-0.2979,0.0147,-0.110231872,0.525103385,214.016806348,0.4321,0.3036,0.5890,0.1128,0.0938,0.0803,0.0956,0.0999,5.2080,0f000001,0*f1eaf58d\n\tsystem status\tnormal 2 27.800000 0 0\trobot status\t31.754396\t41.867619\t9.179500\t-0.110232\t0.525103\t-124.016806\t0.495000\t-0.004000\n\t\n15:51:49.9\tlog_raw\tgps_raw\t#INSPVAXA,USB3,0,45.5,FINESTEERING,2107,283927.950,02000000,471d,15824;INS_ALIGNMENT_COMPLETE,INS_RTKFIXED,37.37050571191,126.72119201313,9.1838,22.3000,-0.3640,-0.2912,0.0308,-0.267249738,0.507353767,214.246041295,0.4321,0.3036,0.5890,0.1128,0.0938,0.0803,0.0956,0.0999,5.2080,0f000001,0*5bacc05f\n\tsystem status\tnormal 2 27.800000 0 0\trobot status\t31.614330\t41.676365\t9.183800\t-0.267250\t0.507354\t-124.246041\t0.493000\t-0.009000\n\t\n15:51:50.4\tlog_raw\tgps_raw\t#INSPVAXA,USB3,0,49.0,FINESTEERING,2107,283928.450,02000000,471d,15824;INS_ALIGNMENT_COMPLETE,INS_RTKFIXED,37.37050398059,126.72119038218,9.1856,22.3000,-0.3631,-0.3028,0.0151,-0.368561001,0.456085807,214.459019955,0.4324,0.3038,0.5890,0.1126,0.0935,0.0802,0.0956,0.0998,5.2095,0f000001,0*73c86a57\n\tsystem status\tnormal 2 27.800000 0 0\trobot status\t31.469863\t41.484216\t9.185600\t-0.368561\t0.456086\t-124.459020\t0.495000\t-0.007000\n\t\n15:51:50.9\tlog_raw\tgps_raw\t#INSPVAXA,USB3,0,49.0,FINESTEERING,2107,283928.950,02000000,471d,15824;INS_ALIGNMENT_COMPLETE,INS_RTKFIXED,37.37050228349,126.72118877638,9.1897,22.3000,-0.3679,-0.3047,0.0058,-0.525199888,0.456229866,214.593983111,0.4324,0.3038,0.5890,0.1126,0.0935,0.0802,0.0956,0.0998,5.2095,0f000001,0*0c17fda2\n
